vi "RT Driver VI.vi"(7 "Operation":T1, 11 "Device Reference in":T2 format="%.0x") -> (0 "Error Code":i32)   [LabVIEW 2017, in "Data Sharing Framework Engine.lvlib"]
uses:
  Data Sharing Framework Engine.lvlib
  VeriStand Framework/VeriStand DSF.Framework.lvclass
  <vilib>/NI Veristand/Custom Device API/Global Data Refs.vi
  <vilib>/NI VeriStand/Custom Device API/Custom Device API.lvlib
  <vilib>/NI Veristand/Custom Device API/Custom Device Item Ref.ctl
  <vilib>/NI Veristand/Custom Device API/Hardware Interface Driver VI Operation.ctl
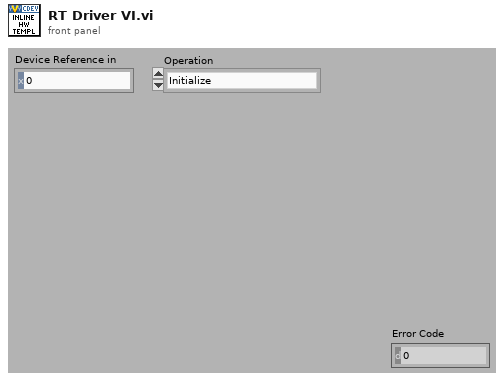
[diagram p1: front panel]
types:
  T1 = typedef "Custom Device API.lvlib/Hardware Interface Driver VI Operation.ctl" = enum16{"Initialize", "Start", "Read Data from HW", "Write Data to HW", "Close"}
  T2 = typedef "Custom Device API.lvlib/Custom Device Item Ref.ctl" = u64
  T3 = typedef "Custom Device API.lvlib/Data Table Ref.ctl" = cluster{"Ptr.Beg":u64, "Ptr.End":u64}
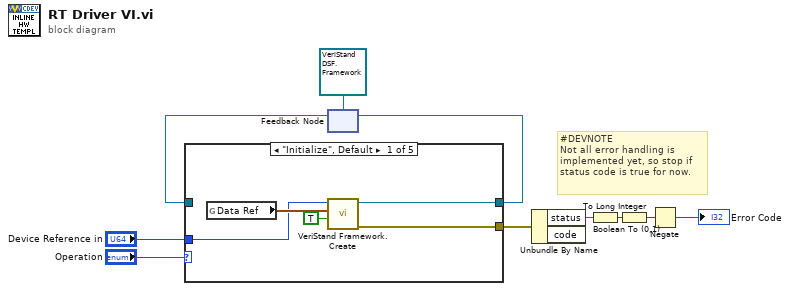
[diagram p0: block diagram]
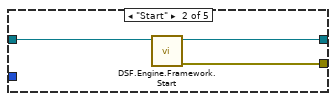
[diagram p2: hidden frame]
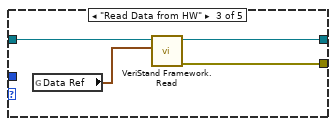
[diagram p3: hidden frame]
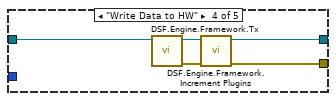
[diagram p4: hidden frame]
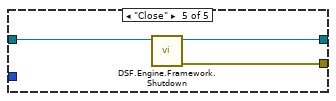
[diagram p5: hidden frame]
diagram:
  # "#DEVNOTE\nNot all error handling is implemented yet, so stop if status code is true for now."
  n1 = feedback #1(refnum<class "VeriStand DSF.Framework.lvclass"> refnum ("Data Sharing Framework Engine.lvlib:VeriStand Framework.lvclass")) -> (w10:refnum<class "VeriStand DSF.Framework.lvclass">)
  n2 = case shown="\"Initialize\", Default" "Operation" {
    tunnel: [w15 w17 w20 w24 w29] -> w7
    tunnel: w10 -> [_ w18 w22 w27 w30]
    tunnel: "Device Reference in" -> [w11 _ _ _ _]
    tunnel: [w14 w16 w21 w23 w28] -> w4
    frame "Initialize", Default {
      n3 = global read "Global Data Refs.vi" "Data Ref"() -> (w13:T3)
      n4 = call "VeriStand Framework.Create.vi"("debug mode (F)"=TRUE, "Engine Data Ref"=w13, "Device Item Ref"=w11) -> ("error out"=w14:errorcluster, "VeriStand Framework out"=w15:refnum<class "VeriStand DSF.Framework.lvclass">)  [unwired: 7 in]
    }
    frame "Start" {
      n5 = call "DSF.Engine.Framework.Start.vi"("Framework in"=w18) -> ("error out"=w16:errorcluster, "Framework out"=w17:refnum<class "VeriStand DSF.Framework.lvclass">)  [unwired: 9 in]
    }
    frame "Read Data from HW" {
      n6 = global read "Global Data Refs.vi" "Data Ref"() -> (w19:T3)
      n7 = call "VeriStand Framework.Read.vi"("Data Ref"=w19, "VeriStand DSF in"=w22) -> ("error out"=w21:errorcluster, "VeriStand DSF out"=w20:refnum<class "VeriStand DSF.Framework.lvclass">)  [unwired: 8 in]
    }
    frame "Write Data to HW" {
      n8 = call "DSF.Engine.Framework.Tx.vi"("Framework in"=w27) -> ("error out"=w25:errorcluster, "Framework out"=w26:refnum<class "VeriStand DSF.Framework.lvclass">)  [unwired: 9 in]
      n9 = call "DSF.Engine.Framework.Increment Plugins.vi"("error in (no error)"=w25, "Framework in"=w26) -> ("error out"=w23:errorcluster, "Framework out"=w24:refnum<class "VeriStand DSF.Framework.lvclass">)  [unwired: 8 in]
    }
    frame "Close" {
      n10 = call "DSF.Engine.Framework.Shutdown.vi"("Framework in"=w30) -> ("error out"=w28:errorcluster, "Framework out"=w29:refnum<class "VeriStand DSF.Framework.lvclass">)  [unwired: 9 in]
    }
  }
  n11 = feedback-in #1(w7) -> ()
  n12 = Unbundle By Name(w4) -> ("status"=w6:bool)  [unwired: 1 out]
  n13 = Boolean To (0,1)(Boolean=w6) -> (0, 1=w5:i16)
  n14 = To Long Integer(number=w5) -> (32bit integer=w2:i32)
  n15 = Negate(x=w2) -> (-x=→"Error Code":i32)
